vi "Create Logic Screen Array.vi"(8 "error in (no error)":errorcluster caption="错误输入（无错误）", 11 "Gif Image 输入":refnum<class "Gif Image.lvclass"> caption="DNL_LabVIEW Object in") -> (0 "error out":errorcluster caption="错误输出", 3 "Gif Image 输出":refnum<class "Gif Image.lvclass"> caption="DNL_LabVIEW Object out")   [LabVIEW 2012, in "Picture Box Tools.lvlib" / "Gif Image.lvclass"]
uses:
  Gif Image.lvclass
  Gif Image.lvclass/Gif Image.ctl
panel:
  in  "BK Color":u32
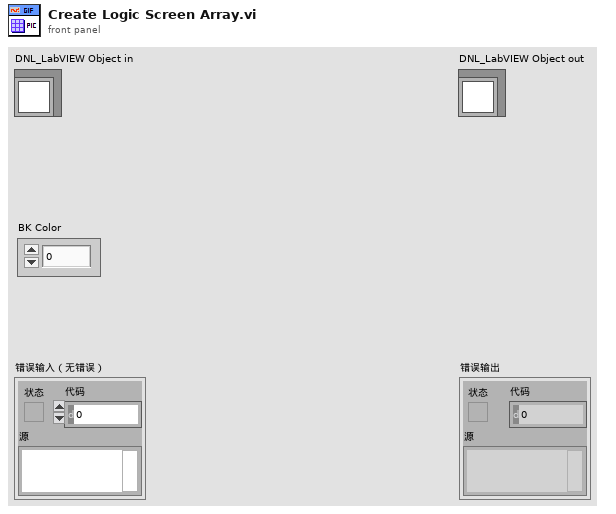
[diagram p1: front panel]
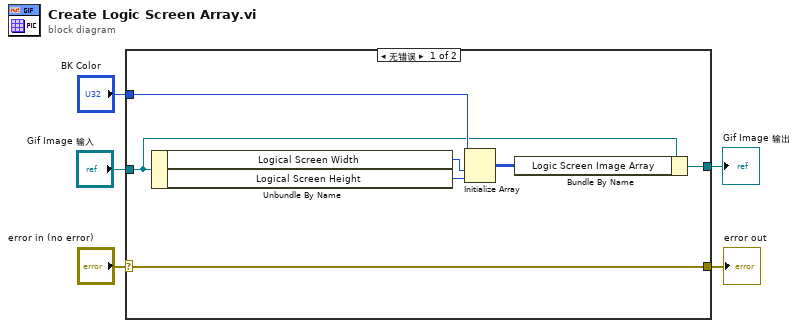
[diagram p0: block diagram]
diagram:
  n1 = case shown="无错误" "error in (no error)" {
    selector: "error in (no error)" -> [w12 w14]
    tunnel: [w12 w14] -> w4
    tunnel: [w6 w13] -> w2
    tunnel: "Gif Image 输入" -> [w8 w13]
    tunnel: "BK Color" -> [w9 _]
    frame No Error {
      n2 = Unbundle By Name(w8) -> ("Logical Screen Width"=w11:u16, "Logical Screen Height"=w10:u16)
      n3 = Initialize Array(w9, w11, w10) -> (w7:u32[][])
      n4 = Bundle By Name(cluster=w8, "Logic Screen Image Array"=w7) -> (w6:refnum<class "Gif Image.lvclass">)
    }
    frame Error {
    }
  }
  "error out" <- w4
  "Gif Image 输出" <- w2
